vi "Write DBL Header.vi"(2 "Error IN":errorcluster, 3 "Physical Lengths (um)":T1, 4 "Pixel Lengths":T2, 5 "File Path IN":path) -> (0 "Error OUT":errorcluster, 1 "File Ref OUT":refnum<file>)   [LabVIEW 2014]
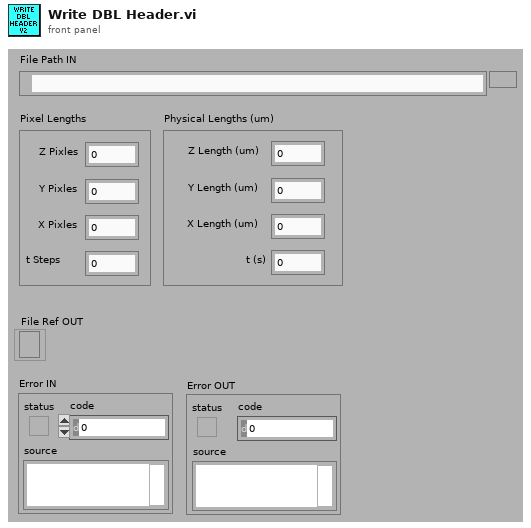
[diagram p1: front panel]
types:
  T1 = cluster{"Z Length (um)":sgl, "Y Length (um)":sgl, "X Length (um)":sgl, "t (s)":sgl}
  T2 = cluster{"Z Pixles":u16, "Y Pixles":u16, "X Pixles":u16, "t Steps":u16}
  T3 = enum16{"big-endian, network order", "native, host order", "little-endian"}
  T4 = enum16{"open", "replace", "create", "open or create", "replace or create", "replace or create with confirmation"}
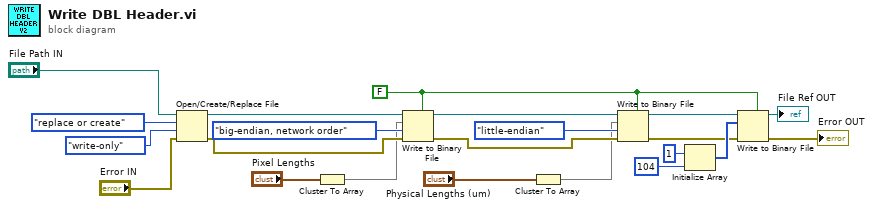
[diagram p0: block diagram]
diagram:
  w11 = FALSE ("prepend array or string size? (T)")
  n1 = Open/Create/Replace File(file path (use dialog)="File Path IN", error in="Error IN", operation (0:open)=T4."replace or create", access (0:read/write)=enum16{"read/write", "read-only", "write-only"}."write-only") -> (refnum out=w20:refnum<file>, error out=w9:errorcluster)  [unwired: 2 in, 1 out]
  n2 = Cluster To Array(cluster="Pixel Lengths") -> (array=w3:u16[])
  n3 = Write to Binary File(file (use dialog)=w20, data=w3, error in=w9, 5:w11, 9:T3."big-endian, network order" ("byte order (0:big-endian, network order)")) -> (refnum out=w17:refnum<file>, error out=w8:errorcluster)  [unwired: 1 in, 1 out]
  n4 = Cluster To Array(cluster="Physical Lengths (um)") -> (array=w2:sgl[])
  n5 = Write to Binary File(file (use dialog)=w17, data=w2, error in=w8, 5:w11, 9:T3."little-endian" ("byte order (0:big-endian, network order)")) -> (refnum out=w12:refnum<file>, error out=w7:errorcluster)  [unwired: 1 in, 1 out]
  n6 = Initialize Array(u8 1 ("element"), 104 ("dimension size")) -> (w10:u8[])
  n7 = Write to Binary File(file (use dialog)=w12, data=w10, error in=w7, 5:w11) -> (refnum out=→"File Ref OUT":refnum<file>, error out=→"Error OUT":errorcluster)  [unwired: 2 in, 1 out]
